vi "UHR-Fleezers Control (host) - 12.0.vi"() -> ()   [LabVIEW 2012] (continued)
            n1096 = Divide(x=w2526, y=w2525) -> (x/y=w2511:dbl[])
            n1097 = Divide(x=w2497, y=w2481) -> (x/y=w2496:dbl[])
            n1098 = Divide(x=w2495, y=w2479) -> (x/y=w2494:dbl[])
            n1099 = Build Array(w2514, w2513, w2528, w2512, w2511, w2525, w2480, w2496, w2481, w2478, w2494, w2479, w2492, w2491) -> (w2490:dbl[][])
            n1100 = Bundle("T1 Y", "T1 X", "T1 Sum", "T2 Y", "T2 X", "T2 Sum", "T1 FB Y", "T1 FB X", "T1 FB Sum", "T2 FB Y", "T2 FB X", "T2 FB Sum", "PSD X", "PSD Y Sum") -> (w2477:T40)  [unwired: 1 out]
            n1101 = To Word Integer(number=w2532) -> (16bit integer=w2476:i16[])
            n1102 = Cluster To Array(cluster=w2477) -> (array=w2523:string[])
          }
        }
      }
    }
    "AI labels" <- w1617
    n1103 = Decimate 1D Array(w1591) -> (w1615:u32[], w1559:u32[])
    n1104 = local read "DMA Update Period (s)"() -> (w1627:dbl)
    n1105 = Build Array(w1615, w1559) -> (w1685:u32[][])
    n1106 = local read "Data Period (s)"() -> (w1465:dbl)
    n1107 = local read "BD 1 Frequency 2 (MHz)"() -> (w1498:dbl)
    n1108 = local read "BD 1 Frequency 1 (MHz)"() -> (w1499:dbl)
    n1109 = Decimate 1D Array(w1506) -> (w1530:i16[], w1529:i16[], w1527:i16[], w1526:i16[])  [unwired: 9 out]
    n1110 = To Double Precision Float(number=w1685) -> (double precision float=w1686:dbl[][])
    n1111 = local read "APD Integration Time (s)"() -> (w1572:dbl)
    n1112 = Multiply(x=w1465, y="Trap Pos. Disp. Downsample") -> (x*y=w1463:dbl)
    n1113 = Divide(x=w1530, y=w1529) -> (x/y=w1531:dbl[])
    n1114 = Divide(x=w1527, y=w1526) -> (x/y=w1528:dbl[])
    n1115 = feedback #6(0.0) -> (w1544:dbl)
    n1116 = Add(x=w1627, y=w1544) -> (x+y=w1725:dbl)
    n1117 = feedback-in #6(w1725) -> ()
    n1118 = local read "AOM X Cal (nm/MHz)"() -> (w1496:dbl)
    n1119 = To Time Stamp(1:w1544) -> (0:w1543:timestamp)
    n1120 = Split 1D Array(array=w1531, index="N El. to Ave.") -> (second subarray=w1534:dbl[])  [unwired: 1 out]
    n1121 = Split 1D Array(array=w1528, index="N El. to Ave.") -> (second subarray=w1533:dbl[])  [unwired: 1 out]
    n1122 = Multiply(x=w1465, y="Trap Disp. Downsample") -> (x*y=w1545:dbl)
    "Display Period (s)" <- w1545
    n1123 = for "Trap AI" {
      tunnel: [w2275] -> w1719 mode=indexing
      tunnel: w1543 -> [w2265]
      tunnel: "Trap Disp. Downsample" -> [w2273]
      tunnel: w1618 -> [w2271] mode=indexing
      tunnel: w1465 -> [w2270]
      tunnel: w1617 -> [w2269] mode=indexing
      tunnel: w1542 -> [w2268]
      tunnel: [w2267] -> w1583 mode=indexing
      tunnel: w1545 -> [w2266]
      workers-P: _ -> [_]
      n1124 = Bundle By Name("Y"=w2271, "dt"=w2270) -> (w2272:waveform(dbl))  [unwired: 1 out]
      n1125 = Set Waveform Attribute(5:w2269, 6:w2268, 7:w2272) -> (3:w2267:waveform(dbl))  [unwired: 1 in, 2 out]
      n1126 = call "downsample 1D array - double.vi"("Ave N"=w2273, "Array In"=w2271) -> ("Array Out"=w2274:dbl[])  [unwired: 1 out]
      n1127 = Bundle By Name(cluster=w2267, "t0"=w2265, "Y"=w2274, "dt"=w2266) -> (w2275:waveform(dbl))
    }
    n1128 = Bundle("BD 1 Frequency 1 (MHz)"=w1499, "BD 1 Frequency 2 (MHz)"=w1498) -> (w1500:T41)  [unwired: 1 out]
    n1129 = call-poly <vilib>:"Mean.vi"("X"=w1533) -> ("mean"=w1521:dbl)  [unwired: 1 out]
    n1130 = call-poly <vilib>:"Mean.vi"("X"=w1534) -> ("mean"=w1522:dbl)  [unwired: 1 out]
    n1131 = Reciprocal(x=w1545) -> (1/x=→"Trap Disp. Freq. (Hz)":dbl)
    n1132 = Cluster To Array(cluster=w1500) -> (array=w1497:dbl[])
    n1133 = local read "Trap X AI1 (DMA)"() -> (w1532:T13)
    n1134 = local read "Data points/scans (MCL)"() -> (w1697:dbl)
    n1135 = To Fixed-Point(number=w1521) -> (fixed-point=w1519:fxp<+/-,16,1>)  [unwired: 1 in]
    n1136 = To Fixed-Point(number=w1522) -> (fixed-point=w1520:fxp<+/-,16,1>)  [unwired: 1 in]
    n1137 = Bundle("Trap 1 Pos.", "Trap 2 Pos.") -> (w1541:cluster{string, string})  [unwired: 1 out]
    n1138 = Bundle By Name(cluster=w1532, "Set 1"=w1520, "Set 2"=w1519) -> (→"Trap X AI1 (DMA)":T13)
    n1139 = Cluster To Array(cluster=w1541) -> (array=w1538:string[])
    n1140 = Bundle("APD 1", "APD 2") -> (w1718:cluster{string, string})  [unwired: 1 out]
    n1141 = Select(t=-1.0, s="Negate Y Axis", f=1.0) -> (s? t:f=w1482:dbl)
    n1142 = for "Trap Position" {
      tunnel: w1547 -> [w1914] mode=indexing
      tunnel: "Trap Pos. Disp. Downsample" -> [w1913]
      tunnel: w1463 -> [w1911]
      tunnel: w1543 -> [w1910]
      tunnel: w1542 -> [w1908]
      tunnel: w1538 -> [w1907] mode=indexing
      tunnel: [w1906] -> w1452 mode=indexing
      tunnel: w1497 -> [w1904] mode=indexing
      tunnel: w1496 -> [w1902]
      tunnel: w1482 -> [w1901]
      n1143 = call "downsample 1D array - double.vi"("Ave N"=w1913, "Array In"=w1914) -> ("Array Out"=w1912:dbl[])  [unwired: 1 out]
      n1144 = Subtract(x=w1912, y=w1904) -> (x-y=w1905:dbl[])
      n1145 = Multiply(x=w1902, y=w1905) -> (x*y=w1903:dbl[])
      n1146 = Multiply(x=w1901, y=w1903) -> (x*y=w1900:dbl[])
      n1147 = Bundle By Name("Y"=w1900, "dt"=w1911, "t0"=w1910) -> (w1909:waveform(dbl))  [unwired: 1 out]
      n1148 = Set Waveform Attribute(5:w1907, 6:w1908, 7:w1909) -> (3:w1906:waveform(dbl))  [unwired: 1 in, 2 out]
    }
    n1149 = Cluster To Array(cluster=w1718) -> (array=w1715:string[])
    n1150 = for "APD" {
      tunnel: w1686 -> [w2254] mode=indexing
      tunnel: w1572 -> [w2262]
      tunnel: [w2258] -> w1579 mode=indexing
      tunnel: "APD Disp. Scale" -> [w2259]
      tunnel: w1542 -> [w2257]
      tunnel: w1715 -> [w2256] mode=indexing
      tunnel: "APD Disp. Downsample" -> [w2252]
      tunnel: [w2255] -> w1714
      workers-P: _ -> [_]
      tunnel: w1543 -> [w2251]
      n1151 = call "integrate 1D array interval - double.vi"("Ave N"=w2252, "Array In"=w2254) -> ("Array Out"=w2253:dbl[])  [unwired: 1 out]
      n1152 = Multiply(x=w2262, y=w2252) -> (x*y=w2255:dbl)
      n1153 = Divide(x=w2253, y=w2259) -> (x/y=w2260:dbl[])
      n1154 = Bundle By Name("t0"=w2251, "Y"=w2260, "dt"=w2255) -> (w2261:waveform(dbl))  [unwired: 1 out]
      n1155 = Set Waveform Attribute(5:w2256, 6:w2257, 7:w2261) -> (3:w2258:waveform(dbl))  [unwired: 1 in, 2 out]
    }
    "APD Display Period (s)" <- w1714
    n1156 = Reciprocal(x=w1714) -> (1/x=→"APD Display Freq. (Hz)":dbl)
    n1157 = local read "Display Period (s)"() -> (w1603:dbl)
    n1158 = Increment(x=w1697) -> (x+1=w1698:dbl)
    n1159 = To Double Precision Float(number=w1615) -> (double precision float=w1614:dbl[])
    n1160 = Index Array(array=w1452, index=0) -> (element=w1456:waveform(dbl))
    n1161 = Index Array(array=w1452, index=1) -> (element=w1451:waveform(dbl))
    n1162 = feedback #7(w1698) -> (w1701:dbl)
    n1163 = Select(t=0, s=w1688, f=w1701) -> (s? t:f=w1694:dbl)
    n1164 = Array Size(array=w1614) -> (size(s)=w1700:i32)
    n1165 = Add(x=w1700, y=w1694) -> (x+y=w1695:dbl)
    n1166 = Unbundle By Name(w1456) -> ("Y"=w1457:dbl[])
    n1167 = feedback #8(w1615) -> (w1684:u32[])
    n1168 = Build Array (concatenate)(w1684, w1615) -> (w1681:u32[])
    n1169 = feedback #9(w1559) -> (w1578:u32[])
    n1170 = Divide(x="Bead Sep. Int. Time (s)", y=w1603) -> (x/y=w1492:dbl)
    n1171 = Build Array (concatenate)(w1578, w1559) -> (w1577:u32[])
    n1172 = Add(x=w1457, y="FB Trap Pos Offset") -> (x+y=w1455:dbl[])
    "T1 x pos data" <- w1455
    n1173 = Greater?(x=w1695, y=w1697) -> (0:w1696:bool)
    n1174 = feedback #10(w1455) -> (w1494:dbl[])
    n1175 = Build Array (concatenate)(w1455, w1494) -> (w1493:dbl[])
    n1176 = Bundle By Name(cluster=w1456, "Y"=w1455) -> (w1454:waveform(dbl))
    n1177 = Select(t=w1694, s=w1696, f=w1695) -> (s? t:f=w1693:dbl)
    n1178 = feedback-in #7(w1693) -> ()
    n1179 = Array Size(array=w1681) -> (size(s)=w1678:i32)
    n1180 = Array Size(array=w1615) -> (size(s)=w1680:i32)
    n1181 = local read "MCL Scanning"() -> (w1691:bool)
    n1182 = local read "APD Integration Time (s)"() -> (w1586:dbl)
    n1183 = Bundle(w1454, w1451) -> (w1450:cluster{waveform(dbl), waveform(dbl)})  [unwired: 1 out]
    n1184 = Build Array (concatenate)(w1579, w1719) -> (w1581:waveform(dbl)[])
    "All Signals" <- w1581
    n1185 = Split 1D Array(array=w1493, index=w1492) -> (first subarray=w1486:dbl[])  [unwired: 1 out]
    n1186 = feedback-in #10(w1486) -> ()
    n1187 = Multiply(x=w1680, y="APD Ave N") -> (x*y=w1679:dbl)
    n1188 = Greater?(x=w1678, y=w1679) -> (0:w1682:bool)
    n1189 = Not(x=w1696) -> (.not. x?=w1690:bool)
    n1190 = Cluster To Array(cluster=w1450) -> (array=w1426:waveform(dbl)[])
    "Trap Positions" <- w1426
    n1191 = To Double Precision Float(number=w1559) -> (double precision float=w1558:dbl[])
    n1192 = call-poly <vilib>:"Mean.vi"("X"=w1486) -> ("mean"=w1485:dbl)  [unwired: 1 out]
    "Mean T1 Position (nm)" <- w1485
    n1193 = Subtract(x=w1486, y=w1485) -> (x-y=w1491:dbl[])
    n1194 = Square(x=w1491) -> (x^2=w1490:dbl[])
    n1195 = And(x=w1690, y=w1691) -> (x .and. y?=w1692:bool)
    n1196 = call-poly <vilib>:"Mean.vi"("X"=w1490) -> ("mean"=w1489:dbl)  [unwired: 1 out]
    n1197 = case shown="True" w1682 {
      tunnel: w1681 -> [w2034 w2041]
      tunnel: [w2034 w2039] -> w1632
      tunnel: w1679 -> [_ w2036]
      tunnel: w1678 -> [_ w2040]
      tunnel: w1577 -> [w2033 w2038]
      tunnel: [w2033 w2035] -> w1574
      frame False {
      }
      frame True {
        n1198 = Subtract(x=w2040, y=w2036) -> (x-y=w2037:dbl)
        n1199 = Array Subset(array=w2041, index=w2037, length=w2036) -> (w2039:u32[])
        n1200 = Array Subset(array=w2038, index=w2037, length=w2036) -> (w2035:u32[])
      }
    }
    n1201 = feedback-in #8(w1632) -> ()
    n1202 = feedback-in #9(w1574) -> ()
    n1203 = Square Root(x=w1489) -> (sqrt(x)=w1488:dbl)
    n1204 = Or(x=w1692, y=w1688) -> (x .or. y?=w1689:bool)
    n1205 = Equal?(x="Tab Control 6", y=T29."High Res Display") -> (x = y?=w1621:bool)
    n1206 = Multiply(x="APD Disp. Scale", y=w1579) -> (x*y=w1588:waveform(dbl)[])
    n1207 = Multiply(x=10.0, y=w1488) -> (x*y=→"Trap 1 Position RMS (A)":dbl)
    n1208 = Multiply(x="APD Disp. Downsample", y=w1586) -> (x*y=w1584:dbl)
    n1209 = Divide(x=w1588, y=w1584) -> (x/y=w1556:waveform(dbl)[])
    n1210 = case "For displaying the high resolution display (no downsampling)" shown="True" w1621 {
      tunnel: w1583 -> [_ w1934]
      frame False {
      }
      frame True {
        n1211 = Index Array(array=w1934, index="High Res. Display") -> (element=w1935:waveform(dbl))
        n1212 = call <vilib>:"Std Deviation and Variance.vi"("X"=w1935) -> ("mean"=w1942:dbl, "standard deviation"=w1947:dbl)  [unwired: 1 in, 1 out]
        "Mean Intensity" <- w1942
        "Sigma" <- w1947
        n1213 = Subtract(x=w1935, y=w1942) -> (x-y=w1941:waveform(dbl))
        n1214 = Select(t=w1941, s="Subtract mean", f=w1935) -> (s? t:f=→"1 Channel":waveform(dbl))
        n1215 = Divide(x=w1947, y=w1942) -> (x/y=→"Sigma/Mean":dbl)
        n1216 = feedback #11(1) -> (w1936:i32)
        n1217 = Greater Or Equal?(x=w1936, y="Slow mean N ave.") -> (x >= y?=w1949:bool)
        n1218 = Increment(x=w1936) -> (x+1=w1951:i32)
        n1219 = Select(t=1, s=w1949, f=w1951) -> (s? t:f=w1938:i32)
        n1220 = feedback-in #11(w1938) -> ()
        n1221 = feedback #12() -> (w1939:waveform(dbl))  [unwired: 1 out]
        n1222 = case shown="Default" w1936 {
          tunnel: [w1954 w1957] -> w1940
          tunnel: w1939 -> [w1956 _]
          tunnel: w1935 -> [w1955 w1957]
          frame Default {
            n1223 = call-poly <vilib>:"Append Waveforms.vi"("waveform B"=w1955, "waveform A"=w1956) -> ("waveform out"=w1954:waveform(dbl))  [unwired: 1 in, 8 out]
          }
          frame 1 {
          }
        }
        n1224 = feedback-in #12(w1940) -> ()
        n1225 = case shown="True" w1949 {
          tunnel: w1940 -> [_ w1953]
          frame False {
          }
          frame True {
            n1226 = call-poly <vilib>:"Mean.vi"("X"=w1953) -> ("mean"=→"Slow mean":dbl)  [unwired: 1 out]
          }
        }
      }
    }
    n1227 = Index Array(array=w1556, index=0) -> (element=w1566:waveform(dbl))
    n1228 = Index Array(array=w1556, index=1) -> (element=w1564:waveform(dbl))
    n1229 = case "For computing FFTs for display" shown="True" "Compute FFT" {
      tunnel: w1583 -> [_ w2648]
      frame False {
      }
      frame True {
        n1230 = Build Array("FFT 1 Choice 1", "FFT 1 Choice 2", "FFT 2 Choice 1", "FFT 2 Choice 2") -> (w2641:u16[])
        n1231 = Array Size(array=w2648) -> (size(s)=w2647:i32)
        n1232 = feedback-in #13(w2641) -> ()
        n1233 = feedback #13(u16[] [100, 100, 100, 100]) -> (w2642:u16[])
        n1234 = feedback-in #14("# Spectra to Ave.") -> ()
        n1235 = feedback #14("# Spectra to Ave.") -> (w2639:dbl)
        n1236 = Not Equal?(x="# Spectra to Ave.", y=w2639) -> (x != y?=w2638:bool)
        n1237 = Not Equal?(x=w2641, y=w2642) -> (x != y?=w2640:bool)
        n1238 = feedback #15(1.0) -> (w2625:dbl)
        n1239 = Compound Arithmetic op=OR("Reset FFT", w2640, w2638) -> (w2623:bool)
        n1240 = Select(t=1.0, s=w2623, f=w2625) -> (s? t:f=w2627:dbl)
        n1241 = Greater?(x=w2627, y="# Spectra to Ave.") -> (0:w2646:bool)
        n1242 = Increment(x=w2627) -> (x+1=w2626:dbl)
        n1243 = feedback-in #15(w2626) -> ()
        n1244 = local read "DMA Update Period (s)"() -> (w2621:dbl)
        n1245 = Multiply(x="# Spectra to Ave.", y=w2621) -> (x*y=→"Ave. Time (s)":dbl)
        n1246 = Build Array(cluster{"f0":dbl, "df":dbl, "magnitude":dbl[]} {"f0"=0.0, "df"=0.0, "magnitude"=[]} ("PSD")) -> (w2630:cluster{"f0":dbl, "df":dbl, "magnitude":dbl[]}[])
        n1247 = Build Array(w2630, w2630, w2630, w2630) -> (w2632:T42)
        n1248 = feedback #16(w2632) -> (w2637:T42)
        n1249 = for {
          N: 4 -> [_]
          tunnel: w2641 -> [w2670] mode=indexing
          tunnel: w2648 -> [w2671]
          tunnel: w2647 -> [w2673]
          tunnel: w2623 -> [w2666]
          tunnel: w2646 -> [w2665]
          tunnel: "# Spectra to Ave." -> [w2664]
          tunnel: [w2663] -> w2636 mode=indexing
          tunnel: w2637 -> [w2668] mode=indexing
          tunnel: [w2667] -> w2624 mode=indexing
          tunnel: w2627 -> [w2662]
          n1250 = Less?(x=w2670, y=w2673) -> (x < y?=w2672:bool)
          n1251 = Index Array(array=w2671, index=w2670) -> (element=w2669:waveform(dbl))
          n1252 = case shown="True" w2672 {
            tunnel: w2669 -> [_ w2690]
            tunnel: w2668 -> [w2675 w2688]
            tunnel: [w2675 w2676] -> w2667
            tunnel: w2666 -> [_ w2687]
            tunnel: w2665 -> [_ w2680]
            tunnel: w2664 -> [_ w2679]
            tunnel: [cluster{"f0":dbl, "df":dbl, "magnitude":dbl[]} {"f0"=0.0, "df"=0.0, "magnitude"=[]} ("PSD") w2681] -> w2663
            tunnel: w2662 -> [_ w2678]
            frame False {
            }
            frame True {
              n1253 = call <vilib>:"Std Deviation and Variance.vi"("X"=w2690) -> ("mean"=w2691:dbl)  [unwired: 1 in, 2 out]
              n1254 = Subtract(x=w2690, y=w2691) -> (x-y=w2689:waveform(dbl))
              n1255 = xnode "Spectral Measurements"("Signals"=w2689) -> ("PSD"=w2683:cluster{"f0":dbl, "df":dbl, "magnitude":dbl[]})  [unwired: 1 in, 1 out]
              n1256 = case shown="False" w2687 {
                tunnel: w2688 -> [w2700 _]
                tunnel: [w2696 w2705] -> w2676
                tunnel: w2683 -> [w2699 w2706]
                tunnel: w2680 -> [w2698 _]
                frame False {
                  n1257 = Build Array (concatenate)(w2700, w2699) -> (w2697:cluster{"f0":dbl, "df":dbl, "magnitude":dbl[]}[])
                  n1258 = case shown="True" w2698 {
                    tunnel: w2697 -> [w2701 w2704]
                    tunnel: [w2701 w2702] -> w2696
                    frame False {
                    }
                    frame True {
                      n1259 = Delete From Array(array=w2704, index=0) -> (array with subset deleted=w2702:cluster{"f0":dbl, "df":dbl, "magnitude":dbl[]}[])  [unwired: 1 in, 1 out]
                    }
                  }
                }
                frame True {
                  n1260 = Build Array(w2706) -> (w2705:cluster{"f0":dbl, "df":dbl, "magnitude":dbl[]}[])
                }
              }
              n1261 = for {
                tunnel: w2676 -> [w2695] mode=indexing
                tunnel: [w2694] -> w2686 mode=indexing
                workers-P: _ -> [_]
                n1262 = Unbundle By Name(w2695) -> ("magnitude"=w2694:dbl[])
              }
              n1263 = Transpose 2D Array(2D array=w2686) -> (transposed array=w2685:dbl[][])
              n1264 = for {
                tunnel: w2685 -> [w2693] mode=indexing
                tunnel: [w2692] -> w2684 mode=indexing
                workers-P: _ -> [_]
                n1265 = Add Array Elements(numeric array=w2693) -> (sum=w2692:dbl)
              }
              n1266 = Select(t=w2679, s=w2680, f=w2678) -> (s? t:f=w2677:dbl)
              n1267 = Divide(x=w2684, y=w2677) -> (x/y=w2682:dbl[])
              n1268 = Bundle By Name(cluster=w2683, "magnitude"=w2682) -> (w2681:cluster{"f0":dbl, "df":dbl, "magnitude":dbl[]})
            }
          }
        }
        n1269 = case shown="True" w2623 {
          tunnel: w2624 -> [w2655 w2661]
          tunnel: [w2655 w2656] -> w2622
          frame False {
          }
          frame True {
            n1270 = Array Subset(array=w2661, index (row)=0 ("index"), length (row)=4 ("length"), index (col)=0 ("index"), length (col)=1 ("length")) -> (w2656:T42)
          }
        }
        n1271 = feedback-in #16(w2622) -> ()
        n1272 = Split 1D Array(array=w2636, index=2) -> (first subarray=→"FFT 1":cluster{"f0":dbl, "df":dbl, "magnitude":dbl[]}[], second subarray=→"FFT 2":cluster{"f0":dbl, "df":dbl, "magnitude":dbl[]}[])
      }
    }
    n1273 = case "For plotting results of scanning MCL" shown="True" w1689 {
      tunnel: w1688 -> [_ w2074]
      tunnel: w1614 -> [_ w2170]
      tunnel: w1697 -> [_ _]
      tunnel: w1583 -> [_ w2144]
      tunnel: w1558 -> [_ w2075]
      tunnel: w1557 -> [_ w2048]
      frame False {
      }
      frame True {
        w2055 = u32 0 items=["Horizontal", "Vertical", "Central", "1st Diagonal", "2nd Diagonal"] ("Type of Symmetry")
        w2083 = u32 0 items=["Horizontal", "Vertical", "Central", "1st Diagonal", "2nd Diagonal"] ("Type of Symmetry")
        w2086 = u32 0 items=["Horizontal", "Vertical", "Central", "1st Diagonal", "2nd Diagonal"] ("Type of Symmetry")
        w2115 = u32 0 items=["Horizontal", "Vertical", "Central", "1st Diagonal", "2nd Diagonal"] ("Type of Symmetry")
        n1274 = Index Array(array=w2144, index=10) -> (element=w2150:waveform(dbl))
        n1275 = Index Array(array=w2144, index=11) -> (element=w2147:waveform(dbl))
        n1276 = local read "Cycles/step (MCL)"() -> (w2100:u64)
        n1277 = Index Array(array=w2144, index="Channel") -> (element=w2146:waveform(dbl))
        n1278 = Unbundle(w2048) -> ("New Image"=w2047:T2, "New Image"=w2046:T2, "New Image"=w2045:T2, "New Image"=w2044:T2)
        n1279 = Unbundle By Name(w2150) -> ("Y"=w2102:dbl[])
        n1280 = Unbundle By Name(w2147) -> ("Y"=w2104:dbl[])
        n1281 = Unbundle By Name(w2146) -> ("Y"=w2109:dbl[])
        n1282 = call "downsample 1D array - double.vi"("Ave N"=w2100, "Array In"=w2102) -> ("Array Out"=w2101:dbl[])  [unwired: 1 out]
        n1283 = call "downsample 1D array - double.vi"("Ave N"=w2100, "Array In"=w2104) -> ("Array Out"=w2103:dbl[])  [unwired: 1 out]
        n1284 = call "downsample 1D array - double.vi"("Ave N"=w2100, "Array In"=w2109) -> ("Array Out"=w2108:dbl[])  [unwired: 1 out]
        n1285 = feedback #17(w2170) -> (w2171:dbl[])
        n1286 = Build Array (concatenate)(w2171, w2170) -> (w2152:dbl[])
        n1287 = feedback #18(w2075) -> (w2077:dbl[])
        n1288 = Build Array (concatenate)(w2077, w2075) -> (w2076:dbl[])
        n1289 = local read "Scan steps (MCL)"() -> (w2057:u64)
        n1290 = Select(t=w2170, s=w2074, f=w2152) -> (s? t:f=w2156:dbl[])
        n1291 = feedback-in #17(w2156) -> ()
        n1292 = Select(t=w2075, s=w2074, f=w2076) -> (s? t:f=w2058:dbl[])
        n1293 = feedback-in #18(w2058) -> ()
        n1294 = local read "Scan lines (y)"() -> (w2043:u64)
        n1295 = local read "N APD Samp/step"() -> (w2059:dbl)
        n1296 = feedback #19(w2101) -> (w2158:dbl[])
        n1297 = Build Array (concatenate)(w2158, w2101) -> (w2149:dbl[])
        n1298 = feedback #20(w2108) -> (w2168:dbl[])
        n1299 = Build Array (concatenate)(w2168, w2108) -> (w2167:dbl[])
        n1300 = feedback #21(w2103) -> (w2160:dbl[])
        n1301 = Build Array (concatenate)(w2160, w2103) -> (w2161:dbl[])
        n1302 = Select(t=w2101, s=w2074, f=w2149) -> (s? t:f=w2105:dbl[])
        n1303 = feedback-in #19(w2105) -> ()
        n1304 = Select(t=w2108, s=w2074, f=w2167) -> (s? t:f=w2107:dbl[])
        n1305 = feedback-in #20(w2107) -> ()
        n1306 = Select(t=w2103, s=w2074, f=w2161) -> (s? t:f=w2106:dbl[])
        n1307 = feedback-in #21(w2106) -> ()
        n1308 = Multiply(x=w2057, y=u64 2) -> (x*y=w2042:u64)
        n1309 = call "integrate 1D array interval - double.vi"("Ave N"=w2059, "Array In"=w2058) -> ("Array Out"=w2070:dbl[])  [unwired: 1 out]
        n1310 = call "integrate 1D array interval - double.vi"("Ave N"=w2059, "Array In"=w2156) -> ("Array Out"=w2155:dbl[])  [unwired: 1 out]
        n1311 = Array Size(array=w2070) -> (size(s)=w2071:i32)
        n1312 = Array Size(array=w2155) -> (size(s)=w2157:i32)
        n1313 = Multiply(x=w2043, y=w2042) -> (x*y=w2073:u64)
        n1314 = Multiply(x=w2043, y=w2042) -> (x*y=w2165:u64)
        n1315 = call-poly <vilib>:"Mean.vi"("X"=w2105) -> ("mean"=w2089:dbl)  [unwired: 1 out]
        n1316 = Subtract(x=w2073, y=w2071) -> (x-y=w2064:u64)
        n1317 = call-poly <vilib>:"Mean.vi"("X"=w2107) -> ("mean"=w2094:dbl)  [unwired: 1 out]
        n1318 = call-poly <vilib>:"Mean.vi"("X"=w2106) -> ("mean"=w2092:dbl)  [unwired: 1 out]
        n1319 = call-poly <vilib>:"Mean.vi"("X"=w2070) -> ("mean"=w2061:dbl)  [unwired: 1 out]
        n1320 = Subtract(x=w2165, y=w2157) -> (x-y=w2099:u64)
        n1321 = call-poly <vilib>:"Mean.vi"("X"=w2155) -> ("mean"=w2096:dbl)  [unwired: 1 out]
        n1322 = Initialize Array(1.0 ("element"), w2064) -> (w2060:dbl[])
        n1323 = Initialize Array(1.0 ("element"), w2099) -> (w2090:dbl[])
        n1324 = Multiply(x=w2060, y=w2061) -> (x*y=w2062:dbl[])
        n1325 = Multiply(x=w2090, y=w2092) -> (x*y=w2093:dbl[])
        n1326 = Multiply(x=w2090, y=w2094) -> (x*y=w2095:dbl[])
        n1327 = Multiply(x=w2090, y=w2089) -> (x*y=w2091:dbl[])
        n1328 = Multiply(x=w2090, y=w2096) -> (x*y=w2097:dbl[])
        n1329 = Build Array (concatenate)(w2105, w2091) -> (w2159:dbl[])
        n1330 = Build Array (concatenate)(w2107, w2095) -> (w2163:dbl[])
        n1331 = Build Array (concatenate)(w2106, w2093) -> (w2162:dbl[])
        n1332 = Build Array (concatenate)(w2070, w2062) -> (w2072:dbl[])
        n1333 = Build Array (concatenate)(w2155, w2097) -> (w2164:dbl[])
        n1334 = Reshape Array(w2159, w2043, w2042) -> (w2125:dbl[][])
        n1335 = Reshape Array(w2072, w2043, w2042) -> (w2068:dbl[][])
        n1336 = Reshape Array(w2163, w2043, w2042) -> (w2117:dbl[][])
        n1337 = Reshape Array(w2162, w2043, w2042) -> (w2132:dbl[][])
        n1338 = Reshape Array(w2164, w2043, w2042) -> (w2142:dbl[][])
        n1339 = Array Subset(array=w2132, index (col)=0 ("index"), length (col)=w2057) -> (w2137:dbl[][])  [unwired: 2 in]
        n1340 = Array Subset(array=w2132, index (col)=w2057) -> (w2135:dbl[][])  [unwired: 3 in]
        n1341 = Array Subset(array=w2117, index (col)=0 ("index"), length (col)=w2057) -> (w2123:dbl[][])  [unwired: 2 in]
        n1342 = Array Subset(array=w2117, index (col)=w2057) -> (w2121:dbl[][])  [unwired: 3 in]
        n1343 = Array Subset(array=w2068, index (col)=0 ("index"), length (col)=w2057) -> (w2067:dbl[][])  [unwired: 2 in]
        n1344 = Array Subset(array=w2068, index (col)=w2057) -> (w2065:dbl[][])  [unwired: 3 in]
        n1345 = Array Subset(array=w2142, index (col)=0 ("index"), length (col)=w2057) -> (w2141:dbl[][])  [unwired: 2 in]
        n1346 = Array Subset(array=w2142, index (col)=w2057) -> (w2139:dbl[][])  [unwired: 3 in]
        n1347 = Array Subset(array=w2125, index (col)=0 ("index"), length (col)=w2057) -> (w2130:dbl[][])  [unwired: 2 in]
        n1348 = Array Subset(array=w2125, index (col)=w2057) -> (w2128:dbl[][])  [unwired: 3 in]
        n1349 = for {
          tunnel: w2137 -> [w2179] mode=indexing
          tunnel: [w2178] -> w2136 mode=indexing
          workers-P: _ -> [_]
          n1350 = Reverse 1D Array(array=w2179) -> (reversed array=w2178:dbl[])
        }
        n1351 = for {
          tunnel: w2123 -> [w2175] mode=indexing
          tunnel: [w2174] -> w2122 mode=indexing
          workers-P: _ -> [_]
          n1352 = Reverse 1D Array(array=w2175) -> (reversed array=w2174:dbl[])
        }
        n1353 = for {
          tunnel: w2067 -> [w2173] mode=indexing
          tunnel: [w2172] -> w2066 mode=indexing
          workers-P: _ -> [_]
          n1354 = Reverse 1D Array(array=w2173) -> (reversed array=w2172:dbl[])
        }
        n1355 = for {
          tunnel: w2141 -> [w2181] mode=indexing
          tunnel: [w2180] -> w2140 mode=indexing
          workers-P: _ -> [_]
          n1356 = Reverse 1D Array(array=w2181) -> (reversed array=w2180:dbl[])
        }
        n1357 = for {
          tunnel: w2130 -> [w2177] mode=indexing
          tunnel: [w2176] -> w2129 mode=indexing
          workers-P: _ -> [_]
          n1358 = Reverse 1D Array(array=w2177) -> (reversed array=w2176:dbl[])
        }
        n1359 = Index Array(array=w2142, index (row)=0) -> (element=→"Waveform Graph":dbl[])  [unwired: 1 in]
        n1360 = Add(x=w2136, y=w2135) -> (x+y=w2134:dbl[][])
        n1361 = Add(x=w2122, y=w2121) -> (x+y=w2120:dbl[][])
        n1362 = Add(x=w2066, y=w2065) -> (x+y=w2050:dbl[][])
        n1363 = Add(x=w2140, y=w2139) -> (x+y=w2114:dbl[][])
        n1364 = Add(x=w2129, y=w2128) -> (x+y=w2127:dbl[][])
        n1365 = Divide(x=w2120, y=2) -> (x/y=w2118:dbl[][])
        n1366 = Divide(x=w2134, y=2) -> (x/y=w2079:dbl[][])
        n1367 = Divide(x=w2127, y=2) -> (x/y=w2081:dbl[][])
        n1368 = To Single Precision Float(number=w2114) -> (single precision float=w2113:sgl[][])
        n1369 = Transpose 2D Array(2D array=w2118) -> (transposed array=→"Data map":dbl[][])
        n1370 = To Single Precision Float(number=w2050) -> (single precision float=w2054:sgl[][])
        n1371 = To Single Precision Float(number=w2079) -> (single precision float=w2085:sgl[][])
        n1372 = To Single Precision Float(number=w2081) -> (single precision float=w2082:sgl[][])
        n1373 = call "IMAQ ArrayToImage"("Image Pixels (Float)"=w2113, "Image"=w2047) -> ("Image Out"=w2116:T2)  [unwired: 8 in, 1 out]
        n1374 = call "IMAQ ArrayToImage"("Image Pixels (Float)"=w2054, "Image"=w2046) -> ("Image Out"=w2056:T2)  [unwired: 8 in, 1 out]
        n1375 = call "IMAQ ArrayToImage"("Image Pixels (Float)"=w2085, "Image"=w2045) -> ("Image Out"=w2087:T2)  [unwired: 8 in, 1 out]
        n1376 = call "IMAQ ArrayToImage"("Image Pixels (Float)"=w2082, "Image"=w2044) -> ("Image Out"=w2084:T2)  [unwired: 8 in, 1 out]
        n1377 = call "IMAQ Symmetry"("Type of Symmetry"=w2115, "Image Src"=w2116) -> ("Image Dst Out"=w2111:T2)  [unwired: 3 in, 1 out]
        n1378 = call "IMAQ Symmetry"("Type of Symmetry"=w2055, "Image Src"=w2056) -> ("Image Dst Out"=w2052:T2)  [unwired: 3 in, 1 out]
        n1379 = call "IMAQ Symmetry"("Type of Symmetry"=w2086, "Image Src"=w2087) -> ("Image Dst Out"=→"Detection Laser X":T2)  [unwired: 3 in, 1 out]
        n1380 = call "IMAQ Symmetry"("Type of Symmetry"=w2083, "Image Src"=w2084) -> ("Image Dst Out"=→"Detection Laser Y":T2)  [unwired: 3 in, 1 out]
        n1381 = call "IMAQ Set Simple Calibration"("Calibration Axis Info"=T30 {"Origin Pixel"={"X"=0.0, "Y"=0.0}, "Angle Relative to Horizontal (deg)"=0.0, "Axis Reference"=0}, "Grid Descriptor"=T31 {"X Step"=0.3, "Y Step"=0.3, "Unit"=enum."Undefined"}, "Image"=w2111) -> ("Calibrated Image"=→"APD 1":T2)  [unwired: 7 in, 1 out]
        n1382 = call "IMAQ Set Simple Calibration"("Calibration Axis Info"=T30 {"Origin Pixel"={"X"=0.0, "Y"=0.0}, "Angle Relative to Horizontal (deg)"=0.0, "Axis Reference"=0}, "Grid Descriptor"=T31 {"X Step"=0.3, "Y Step"=0.3, "Unit"=enum."Undefined"}, "Image"=w2052) -> ("Calibrated Image"=→"APD 2":T2)  [unwired: 7 in, 1 out]
      }
    }
    n1383 = Subtract(x=w1564, y="APD 2 Offset") -> (x-y=w1561:waveform(dbl))
    n1384 = Subtract(x=w1566, y="APD 1 Offset") -> (x-y=w1562:waveform(dbl))
    n1385 = Index Array(array=w1581, index=3) -> (element=w1641:waveform(dbl))
    n1386 = Index Array(array=w1581, index=6) -> (element=w1638:waveform(dbl))
    n1387 = Build Array(w1562, w1561) -> (→"APD Chart":waveform(dbl)[])
    n1388 = Array Size(array=w1632) -> (size(s)=w1677:i32)
    n1389 = call <vilib>:"Std Deviation and Variance.vi"("X"=w1574) -> ("standard deviation"=w1573:dbl)  [unwired: 1 in, 2 out]
    n1390 = Add Array Elements(numeric array=w1574) -> (sum=w1576:u32)
    n1391 = Add Array Elements(numeric array=w1632) -> (sum=w1687:u32)
    n1392 = call <vilib>:"Std Deviation and Variance.vi"("X"=w1632) -> ("standard deviation"=w1631:dbl)  [unwired: 1 in, 2 out]
    n1393 = Divide(x="T1 offset_x (mV)", y=1000.0) -> (x/y=w1642:dbl)
    n1394 = Divide(x=w1573, y=w1572) -> (x/y=w1569:dbl)
    "Rate sigma (Hz) 2" <- w1569
    n1395 = Multiply(x=w1572, y=w1677) -> (x*y=w1575:dbl)
    "Int. Time (s)" <- w1575
    n1396 = Divide(x=w1576, y=w1575) -> (x/y=w1570:dbl)
    "APD 2 Rate (Hz)" <- w1570
    n1397 = Divide(x=w1687, y=w1575) -> (x/y=w1629:dbl)
    "APD 1 Rate (Hz)" <- w1629
    n1398 = Divide(x=w1631, y=w1572) -> (x/y=w1630:dbl)
    "Rate sigma (Hz)" <- w1630
    n1399 = Divide(x=w1569, y=w1570) -> (x/y=→"Sigma/Mean 2":dbl)
    n1400 = Divide(x=w1630, y=w1629) -> (x/y=→"Sigma/Mean":dbl)
    n1401 = feedback-in #22("Calibration") -> ()
    n1402 = feedback #22(u16 1 ("Calibration")) -> (w1660:u16)
    n1403 = Divide(x="T2 offset_x (mV)", y=1000.0) -> (x/y=w1640:dbl)
    n1404 = case shown="0, Default" "Calibration" {
      tunnel: "T1 alpha_x (nm/V)" -> [_ w2010 w2031]
      tunnel: "T1 kappa_x (pN/nm)" -> [_ _ w2021]
      tunnel: "T2 alpha_x (nm/V)" -> [_ w2009 w2029]
      tunnel: "T2 kappa_x (pN/nm)" -> [_ _ w2022]
      tunnel: w1641 -> [w1992 w2007 w2027]
      tunnel: w1638 -> [w1991 w2005 w2025]
      tunnel: [w1992 w2004 w2024] -> w1669
      tunnel: [w1991 w2003 w2023] -> w1668
      tunnel: ["T1 X (V)" ("Label.Text") "T1 X (nm)" ("Label.Text") "T1 X (pN)" ("Label.Text")] -> w1657
      tunnel: ["T2 X (V)" ("Label.Text") "T2 X (nm)" ("Label.Text") "T2 X (pN)" ("Label.Text")] -> w1656
      tunnel: ["Position (V)" ("Label.Text") "Position (nm)" ("Label.Text") "Force (pN)" ("Label.Text")] -> w1658
      tunnel: w1640 -> [_ w1995 w2014]
      tunnel: w1642 -> [_ w1998 w2016]
      tunnel: ["Mean (V)" ("Label.Text") "Mean (nm)" ("Label.Text") "Mean (pN)" ("Label.Text")] -> w1653
      tunnel: ["Difference (V)" ("Label.Text") "Difference (nm)" ("Label.Text") "Difference (pN)" ("Label.Text")] -> w1589
      frame 0, Default {
      }
      frame 1 {
        n1405 = Unbundle By Name(w2007) -> ("Y"=w2011:dbl[])
        n1406 = Unbundle By Name(w2005) -> ("Y"=w1996:dbl[])
        n1407 = Subtract(x=w2011, y=w1998) -> (x-y=w1999:dbl[])
        n1408 = Subtract(x=w1996, y=w1995) -> (x-y=w1997:dbl[])
        n1409 = Multiply(x=w1997, y=w2009) -> (x*y=w2006:dbl[])
        n1410 = Multiply(x=w2010, y=w1999) -> (x*y=w2008:dbl[])
        n1411 = Bundle By Name(cluster=w2005, "Y"=w2006) -> (w2003:waveform(dbl))
        n1412 = Bundle By Name(cluster=w2007, "Y"=w2008) -> (w2004:waveform(dbl))
      }
      frame 2 {
        n1413 = Unbundle By Name(w2027) -> ("Y"=w2032:dbl[])
        n1414 = Unbundle By Name(w2025) -> ("Y"=w2030:dbl[])
        n1415 = Subtract(x=w2030, y=w2014) -> (x-y=w2015:dbl[])
        n1416 = Subtract(x=w2032, y=w2016) -> (x-y=w2017:dbl[])
        n1417 = Compound Arithmetic op=MULTIPLY(w2015, w2029, w2022) -> (w2026:dbl[])
        n1418 = Compound Arithmetic op=MULTIPLY(w2021, w2031, w2017) -> (w2028:dbl[])
        n1419 = Bundle By Name(cluster=w2025, "Y"=w2026) -> (w2023:waveform(dbl))
        n1420 = Bundle By Name(cluster=w2027, "Y"=w2028) -> (w2024:waveform(dbl))
      }
    }
    n1421 = Not Equal?(x=w1660, y="Calibration") -> (x != y?=w1619:bool)
    n1422 = case shown="True" w1619 {
      tunnel: w1658 -> [_ w1985]
      tunnel: w1657 -> [_ w1984]
      tunnel: w1656 -> [_ w1983]
      tunnel: w1653 -> [_ w1982]
      tunnel: w1589 -> [_ w1981]
      frame False {
      }
      frame True {
        n1423 = property on="Force" class="WFChart (strict)"("YScale.NameLbl.Text"=w1985) -> ()  [unwired: 2 in, 2 out]
        n1424 = property on="T2 X" class="DigNum (strict)"("Caption.Text"=w1983) -> ()  [unwired: 2 in, 2 out]
        n1425 = property on="T1 X" class="DigNum (strict)"("Caption.Text"=w1984) -> ()  [unwired: 2 in, 2 out]
        n1426 = property on="Mean" class="DigNum (strict)"("Caption.Text"=w1982) -> ()  [unwired: 2 in, 2 out]
        n1427 = property on="Difference" class="DigNum (strict)"("Caption.Text"=w1981) -> ()  [unwired: 2 in, 2 out]
      }
    }
    n1428 = Unbundle By Name(w1641) -> ("Y"=w1644:dbl[])
    n1429 = Unbundle By Name(w1638) -> ("Y"=w1647:dbl[])
    n1430 = Subtract(x=w1644, y=w1642) -> (x-y=w1645:dbl[])
    n1431 = Subtract(x=w1647, y=w1640) -> (x-y=w1646:dbl[])
    n1432 = Multiply(x=w1646, y="T2 alpha_x (nm/V)") -> (x*y=w1431:dbl[])
    n1433 = Multiply(x="T1 alpha_x (nm/V)", y=w1645) -> (x*y=w1432:dbl[])
    n1434 = Not(x="Trap Trig. Fl.") -> (.not. x?=w1468:bool)
    n1435 = Multiply(x=w1668, y=-1.0) -> (x*y=w1649:waveform(dbl))
    n1436 = Subtract(x=w1432, y=w1431) -> (x-y=w1637:dbl[])
    n1437 = Unbundle By Name(w1668) -> ("Y"=w1608:dbl[])
    n1438 = Unbundle By Name(w1669) -> ("Y"=w1433:dbl[])
    n1439 = Negate(x=w1637) -> (-x=w1429:dbl[])
    n1440 = Build Array(w1669, w1649) -> (→"Force":waveform(dbl)[])
    n1441 = Subtract(x=w1429, y="Offset (nm)") -> (x-y=w1606:dbl[])
    n1442 = case shown="True" "Read Lateness and Rel Phase" {
      tunnel: w1449 -> [w1958 w1980]
      tunnel: w1448 -> [w1959 w1979]
      tunnel: [w1958 w1978] -> w1635
      tunnel: [w1959 w1977] -> w1634
      frame False {
      }
      frame True {
        n1443 = xnode "Read/Write Control"("FPGA VI Reference In"=w1980, "error in"=w1979) -> ("FPGA VI Reference Out"=w1978:T19, "error out"=w1977:errorcluster, "GI Relative phase"=→"GI relative phase":i16, "Relative phase"=→"Relative phase (AI1)":i16, "AI Late Counter"=→"Late Counter (AI1)":u16, "GI Late Counter"=→"GI Late Counter":u16, "MCL Late Counter"=→"MCL Late Counter":u16, "MCL Relative Phase"=→"Relative Phase (MCL)":i16, "APD Acq Relative Phase"=→"APD Acq Relative Phase":i16, "APD 1 Gate Relative Phase"=→"APD 1 Gate Relative Phase":i16, "APD 2 Gate Relative Phase"=→"APD 2 Gate Relative Phase":i16, "APD Acq Late Counter"=→"APD Acq Late Counter":u16, "APD 1 Gate Late Counter"=→"APD 1 Gate Late Counter":u16, "APD 2 Gate Late Counter"=→"APD 2 Gate Late Counter":u16, "Green FB Relative Phase"=→"Relative phase (Green FB)":i16, "GI Relative phase 2"=→"GI relative phase 2":i16, "GI Late Counter 2"=→"GI Late Counter 2":u16, "Trap Pos FIFO Timeout"=→"Trap Pos FIFO Timeout":u16, "Trap AI FIFO Timeout"=→"Trap AI FIFO Timeout":u16)
      }
    }
    n1444 = call-poly <vilib>:"Mean.vi"("X"=w1608) -> ("mean"=w1435:dbl)  [unwired: 1 out]
    "T2 X" <- w1435
    n1445 = Negate(x=w1608) -> (-x=w1609:dbl[])
    n1446 = call-poly <vilib>:"Mean.vi"("X"=w1433) -> ("mean"=w1436:dbl)  [unwired: 1 out]
    "T1 X" <- w1436
    n1447 = Negate(x=w1435) -> (-x=w1434:dbl)
    n1448 = Bundle By Name(cluster=w1641, "Y"=w1606) -> (w1580:waveform(dbl))
    "Bead Separation" <- w1580
    n1449 = Add(x=w1433, y=w1609) -> (x+y=w1610:dbl[])
    n1450 = Add(x=w1436, y=w1434) -> (x+y=w1655:dbl)
    n1451 = Subtract(x=w1436, y=w1434) -> (x-y=→"Difference":dbl)
    n1452 = Divide(x=w1610, y=2.0) -> (x/y=→"Vec Mean of T1 T2":dbl[])
    n1453 = Divide(x=w1655, y=2.0) -> (x/y=w1612:dbl)
    "Mean" <- w1612
    n1454 = feedback-in #23("Trap Trig. Fl.") -> ()
    n1455 = feedback #23("Trap Trig. Fl.") -> (w1466:bool)
    n1456 = And(x=w1468, y=w1466) -> (x .and. y?=w1467:bool)
    n1457 = case "If have just turned off triggering" shown="True" w1467 {
      tunnel: w1449 -> [_ w1793]
      tunnel: w1448 -> [_ w1792]
      frame False {
      }
      frame True {
        w1791 = FALSE ("FPGA Trap Trig")
        n1458 = xnode "Read/Write Control"("FPGA VI Reference In"=w1793, "error in"=w1792, "FPGA Trap Trig"=w1791) -> ("FPGA VI Reference Out"=w1790:T19, "error out"=w1789:errorcluster)
        n1459 = xnode "Read/Write Control"("FPGA VI Reference In"=w1790, "error in"=w1789, "TTrig?"=w1791) -> ()  [unwired: 2 out]
        n1460 = local write "Initializing"(FALSE ("Initializing")) -> ()
        n1461 = local write "Triggered"(FALSE ("Triggered")) -> ()
        n1462 = local write "Waiting"(FALSE ("Waiting")) -> ()
      }
    }
    n1463 = Not(x=w1466) -> (.not. x?=w1479:bool)
    n1464 = And(x="Trap Trig. Fl.", y=w1479) -> (x .and. y?=w1476:bool)
    n1465 = local read "Tether"() -> (w1613:bool)
    n1466 = Or(x=w1476, y="Reinitialize") -> (x .or. y?=w1462:bool)
    n1467 = feedback #24(w1472) -> (w1477:string)
    n1468 = Select(t=w1472, s=w1476, f=w1477) -> (s? t:f=w1471:string)
    n1469 = Select(t=w1472, s="Reinitialize", f=w1471) -> (s? t:f=w1470:string)
    n1470 = feedback #25(0) -> (w1474:i32)
    n1471 = feedback #26(w1606) -> (w1605:dbl[])
    n1472 = Build Array (concatenate)(w1606, w1605) -> (w1430:dbl[])
    n1473 = case "For determining if there is a tether still" shown="True" w1613 {
      tunnel: w1612 -> [_ w1917]
      frame False {
      }
      frame True {
        n1474 = Greater?(x="Lost Tether Alarm Threshold (pN)", y=w1917) -> (0:w1915:bool)
        n1475 = case shown="True" w1915 {
          frame False {
          }
          frame True {
            w1918 = FALSE ("Value (Signaling)")
            n1476 = flat-sequence {
              frame #0 {
                # "stop only if saving"
                n1477 = local read "Saving..."() -> (w1930:bool)
                n1478 = And(x=w1930, y="TA Cancel Save?") -> (x .and. y?=w1929:bool)
                n1479 = local write "Stop Saving"(w1929) -> ()
              }
              frame #1 {
                n1480 = case shown="True" "TA Green Off?" {
                  frame False {
                  }
                  frame True {
                    w1933 = FALSE ("Fl. Triggered...")
                    n1481 = local write "Fl. Triggered..."(w1933) -> ()
                    n1482 = property on="Green Laser ON/Interlacing" class="Bool (strict)"("Val(Sgnl)"=w1933) -> ()  [unwired: 2 in, 2 out]
                  }
                }
              }
            }
            n1483 = local read "Time tether formed"() -> (w1924:timestamp)
            n1484 = Get Date/Time In Seconds() -> (seconds since 1Jan1904=w1925:timestamp)
            n1485 = Subtract(x=w1925, y=w1924) -> (x-y=w1923:dbl)
            n1486 = Number To Decimal String(number=w1923) -> (decimal integer string=w1920:string)  [unwired: 1 out]
            n1487 = local read "Messages"() -> (w1927:string)
            n1488 = call <vilib>:"Beep.vi"() -> ()  [unwired: 3 in, 9 out]
            n1489 = Concatenate Strings("Lost tether (" ("Message to add"), w1920, " s)." ("string")) -> (w1922:string)
            n1490 = local write "Tether"(FALSE ("Tether")) -> ()
            n1491 = call "Update messages.vi"("Message to add"=w1922, "Old message string"=w1927) -> ("New message string"=w1926:string)
            n1492 = local write "Messages"(w1926) -> ()
            n1493 = property on="Fl. Triggered..." class="Bool (strict)"("Val(Sgnl)"=w1918) -> ()  [unwired: 2 in, 2 out]
            n1494 = local write "Dip for Protein"(w1918) -> ()
            n1495 = property on="Trap Pos. FB ON" class="Bool (strict)"("Val(Sgnl)"=w1918) -> ()  [unwired: 2 in, 2 out]
            n1496 = property on="Trap Trig. Fl." class="Bool (strict)"("Val(Sgnl)"=w1918) -> ()  [unwired: 2 in, 2 out]
          }
        }
      }
    }
    n1497 = case "For triggering actions based on the trap position (e.g., turning the excitation laser on if trap under feedback moves so far)" shown="True" "Trap Trig. Fl." {
      tunnel: w1457 -> [_ w1806]
      tunnel: w1470 -> [_ w1805]
      tunnel: ["" ("t") w1804] -> w1478
      tunnel: w1462 -> [_ w1803]
      tunnel: [0 ("t") w1802] -> w1475
      tunnel: w1474 -> [_ w1801]
      tunnel: w1449 -> [_ w1800]
      tunnel: w1448 -> [_ w1799]
      frame False {
      }
      frame True {
        n1498 = case shown="\"Wait for trigger\"" w1805 {
          tunnel: w1806 -> [w1823 _ _ w1871]
          tunnel: [w1820 w1852 "" ("t") w1874] -> w1804
          tunnel: w1803 -> [_ _ _ w1862]
          tunnel: [w1819 w1849 0 ("t") w1863] -> w1802
          tunnel: w1801 -> [_ w1851 _ w1869]
          tunnel: w1800 -> [w1808 w1846 _ w1865]
          tunnel: w1799 -> [w1807 w1845 _ w1864]
          frame "Wait for trigger" {
            n1499 = local read "Trap Trig. (FPGA)"() -> (w1811:bool)
            n1500 = Subtract(x=w1823, y="Mean T1 Position\nto compare (nm)") -> (x-y=w1816:dbl[])
            n1501 = call <vilib>:"Std Deviation and Variance.vi"("X"=w1816) -> ("mean"=→"mean":dbl, "standard deviation"=→"standard\ndeviation":dbl)  [unwired: 1 in, 1 out]
            n1502 = Array Max & Min(array=w1816) -> (max value=→"max value":dbl, min value=→"min value":dbl)  [unwired: 2 out]
            n1503 = Greater?(x=w1816, y="Threshold (nm)") -> (0:w1826:bool[])
            n1504 = case shown="True" w1811 {
              tunnel: w1808 -> [_ w1832]
              tunnel: w1807 -> [_ w1831]
              tunnel: [FALSE ("TTrig?") w1830] -> w1814
              frame False {
              }
              frame True {
                n1505 = xnode "Read/Write Control"("FPGA VI Reference In"=w1832, "error in"=w1831) -> ("TTrig?"=w1830:bool)  [unwired: 2 out]
              }
            }
            n1506 = Or Array Elements(Boolean array=w1826) -> (logical OR=w1813:bool)
            n1507 = Select(t=w1814, s=w1811, f=w1813) -> (s? t:f=w1812:bool)
            n1508 = Not(x=w1811) -> (.not. x?=w1810:bool)
            n1509 = And(x=w1812, y=w1810) -> (x .and. y?=w1809:bool)
            n1510 = Select(t="Triggered", s=w1812, f="Wait for trigger") -> (s? t:f=w1820:string)
            n1511 = case shown="True" w1812 {
              tunnel: [0 0] -> w1819
              tunnel: w1808 -> [_ w1837]
              tunnel: w1807 -> [_ w1836]
              frame False {
                "Waiting" <- TRUE ("Waiting")
              }
              frame True {
                n1512 = xnode "Read/Write Control"("FPGA VI Reference In"=w1837, "error in"=w1836, "TTrig?"=FALSE) -> ()  [unwired: 2 out]
                n1513 = local read "Messages"() -> (w1840:string)
                n1514 = call <vilib>:"Beep.vi"() -> ()  [unwired: 12 in]
                n1515 = call "Update messages.vi"("Message to add"="Unwinding trigger.", "Old message string"=w1840) -> ("New message string"=w1841:string)
                n1516 = local write "Messages"(w1841) -> ()
                n1517 = local write "Waiting"(FALSE ("Waiting")) -> ()
                "Triggered" <- TRUE ("Triggered")
              }
            }
            n1518 = case "Only need to turn on laser if host triggered" shown="True" w1809 {
              frame False {
              }
              frame True {
                n1519 = property on="Green Laser ON/Interlacing" class="Bool (strict)"("Val(Sgnl)"=TRUE ("Value (Signaling)")) -> ()  [unwired: 2 in, 2 out]
              }
            }
          }
          frame "Triggered" {
            n1520 = local read "Trap Trig. (FPGA)"() -> (w1848:bool)
            n1521 = Increment(x=w1851) -> (x+1=w1849:i32)
            n1522 = Greater Or Equal?(x=w1849, y="Fl. ON time (n)") -> (x >= y?=w1847:bool)
            n1523 = Select(t="Wait for trigger", s=w1847, f="Triggered" ("t")) -> (s? t:f=w1852:string)
            n1524 = And(x=w1847, y=w1848) -> (x .and. y?=w1844:bool)
            n1525 = case shown="True" w1844 {
              tunnel: w1846 -> [_ w1856]
              tunnel: w1845 -> [_ w1855]
              frame False {
              }
              frame True {
                n1526 = xnode "Read/Write Control"("FPGA VI Reference In"=w1856, "error in"=w1855, "FPGA Trap Trig"=TRUE) -> ()  [unwired: 2 out]
              }
            }
            n1527 = case shown="True" w1847 {
              frame False {
              }
              frame True {
                w1858 = FALSE ("Value (Signaling)")
                n1528 = local write "Triggered"(w1858) -> ()
                n1529 = local write "Waiting"(TRUE ("Waiting")) -> ()
                n1530 = property on="Green Laser ON/Interlacing" class="Bool (strict)"("Val(Sgnl)"=w1858) -> ()  [unwired: 2 in, 2 out]
              }
            }
          }
          frame "Do nothing" {
          }
          frame "Initialize", Default {
            n1531 = Increment(x=w1869) -> (x+1=w1873:i32)
            n1532 = Select(t=1, s=w1862, f=w1873) -> (s? t:f=w1863:i32)
            n1533 = feedback #27(w1871) -> (w1877:dbl[])
            n1534 = Build Array (concatenate)(w1871, w1877) -> (w1870:dbl[])
            n1535 = Greater Or Equal?(x=w1863, y="Wait to get offset (n)") -> (x >= y?=w1866:bool)
            n1536 = Select(t=w1871, s=w1862, f=w1870) -> (s? t:f=w1872:dbl[])
            n1537 = feedback-in #27(w1872) -> ()
            n1538 = call-poly <vilib>:"Mean.vi"("X"=w1872) -> ("mean"=w1867:dbl)  [unwired: 1 out]
            n1539 = local write "Mean T1 Position\nto compare (nm)"(w1867) -> ()
            n1540 = case shown="True" w1862 {
              tunnel: w1865 -> [_ w1883]
              tunnel: w1864 -> [_ w1882]
              frame False {
              }
              frame True {
                w1879 = FALSE ("FPGA Trap Trig")
                n1541 = xnode "Read/Write Control"("FPGA VI Reference In"=w1883, "error in"=w1882, "FPGA Trap Trig"=w1879) -> ("FPGA VI Reference Out"=w1881:T19, "error out"=w1880:errorcluster)
                n1542 = xnode "Read/Write Control"("FPGA VI Reference In"=w1881, "error in"=w1880, "TTrig?"=w1879) -> ()  [unwired: 2 out]
              }
            }
            n1543 = Select(t="Wait for trigger", s=w1866, f="Initialize") -> (s? t:f=w1874:string)
            n1544 = case shown="True" w1866 {
              tunnel: w1867 -> [_ w1886]
              tunnel: w1865 -> [_ w1895]
              tunnel: w1864 -> [_ w1894]
              frame False {
                n1545 = local write "Waiting"(FALSE ("Waiting")) -> ()
                "Initializing" <- TRUE ("Initializing")
              }
              frame True {
                n1546 = local read "Threshold (nm)"() -> (w1898:dbl)
                n1547 = local read "AOM X Cal (nm/MHz)"() -> (w1897:dbl)
                n1548 = Add(x=w1886, y=w1898) -> (x+y=w1899:dbl)
                n1549 = Divide(x=w1899, y=w1897) -> (x/y=w1896:dbl)
                n1550 = call "IR AOM freq to word.vi"("Frequency In (MHz)"=w1896) -> ("Frequency Word Out (double)"=w1893:dbl)
                n1551 = local write "Initializing"(FALSE ("Initializing")) -> ()
                n1552 = local write "Waiting"(TRUE ("Waiting")) -> ()
                n1553 = To Quad Integer(1:w1893) -> (0:w1892:i64)
                n1554 = xnode "Read/Write Control"("FPGA VI Reference In"=w1895, "error in"=w1894, "FPGA TTrig Thresh"=w1892) -> ("FPGA VI Reference Out"=w1889:T19, "error out"=w1888:errorcluster)
                n1555 = xnode "Read/Write Control"("FPGA VI Reference In"=w1889, "error in"=w1888, "FPGA Trap Trig"=TRUE) -> ()  [unwired: 2 out]
              }
            }
          }
        }
      }
    }
    n1556 = feedback-in #24(w1478) -> ()
    n1557 = feedback-in #25(w1475) -> ()
    n1558 = Split 1D Array(array=w1430, index=w1492) -> (first subarray=w1602:dbl[])  [unwired: 1 out]
    n1559 = feedback-in #26(w1602) -> ()
    n1560 = call-poly <vilib>:"Mean.vi"("X"=w1602) -> ("mean"=w1601:dbl)  [unwired: 1 out]
    "Bead Mean (nm)" <- w1601
    n1561 = Subtract(x=w1602, y=w1601) -> (x-y=w1600:dbl[])
    n1562 = Square(x=w1600) -> (x^2=w1599:dbl[])
    n1563 = call-poly <vilib>:"Mean.vi"("X"=w1599) -> ("mean"=w1598:dbl)  [unwired: 1 out]
    n1564 = Square Root(x=w1598) -> (sqrt(x)=w1597:dbl)
    n1565 = Multiply(x=10.0, y=w1597) -> (x*y=→"RMS (Ang)":dbl)
    n1566 = xnode ("Read/Write Control")("FPGA VI Reference In"=w1635, "error in"=w1634) -> ("FPGA VI Reference Out"=w1460:T19, "error out"=w1459:errorcluster, "AI2 Y Sum Set 1"=w1733:i16, "AI2 Y Sum Set 2"=w1732:i16, "AI1 X Set 1"=w1524:fxp<+/-,16,1>, "AI1 X Set 2"=w1523:fxp<+/-,16,1>, "Trap Pos FB Int Signal"=→"Trap Pos FB Int Signal":fxp<+/-,24,9>, "Trap Pos FB Int-Norm Signal"=→"Trap Pos FB Int-Norm Signal":fxp<+/-,16,1>, "Trap Pos FB Action"=w1517:i64, "Scanning"=→"AOD Scanning":bool, "Scan I"=→"AOD Scan I":u64, "Scanning MCL"=w1735:bool, "Scan I (MCL)"=→"MCL Scan I":u64, "Green FB Sum"=w1672:i16, "Trap Pos FB Action"=w1447:i64, "TTrig Fin Thresh"=w1443:i64)
    "MCL Scanning" <- w1735
    "Trap Pos FB Action" <- w1517
    n1567 = local read "FB Trig Integrate"() -> (w1441:u32)
    n1568 = Divide(x=w1672, y=3276.7) -> (x/y=→"Green laser plot" →"Green laser intensity (V)":dbl)
    n1569 = Divide(x=w1447, y=w1441) -> (x/y=w1440:dbl)
    "TTrig Sig (Int)" <- w1440
    n1570 = Divide(x=w1443, y=w1441) -> (x/y=w1438:dbl)
    "TTrig Fin Thresh (Int)" <- w1438
    n1571 = local read "AOM X Cal (nm/MHz)"() -> (w1446:dbl)
    n1572 = local read "AI2 (V)"() -> (w1734:cluster{"Set 1":dbl, "Set 2":dbl})
    n1573 = Bundle By Name(cluster=w1734, "Set 1"=w1733, "Set 2"=w1732) -> (w1730:cluster{"Set 1":dbl, "Set 2":dbl})
    n1574 = Divide(x=w1517, y=327.67) -> (x/y=→"Action (%)":dbl)
    n1575 = local read "Trap X (AI1)"() -> (w1537:T10)
    n1576 = call "IR AOM word double to freq.vi"("Frequency Word In (double)"=w1438) -> ("Frequency Out (MHz)"=w1437:dbl)
    n1577 = call "IR AOM word double to freq.vi"("Frequency Word In (double)"=w1440) -> ("Frequency Out (MHz)"=w1439:dbl)
    n1578 = Divide(x=w1730, y=3276.7) -> (x/y=w1729:cluster{"Set 1":dbl, "Set 2":dbl})
    n1579 = Multiply(x=w1439, y=w1446) -> (x*y=w1445:dbl)
    "TTrig Sig (nm)" <- w1445
    n1580 = Multiply(x=w1437, y=w1446) -> (x*y=w1444:dbl)
    "TTrig Fin Thresh (nm)" <- w1444
    n1581 = local write "AI2 (V)"(w1729) -> ()
    n1582 = Bundle(cluster=w1537, "Trap 1"=w1524, "Trap 2"=w1523) -> (→"Trap X (AI1)":T10)
    n1583 = Bundle(w1445, w1444) -> (→"TTrig":cluster{dbl, dbl})  [unwired: 1 in]
    n1584 = flat-sequence "To save data" {
      tunnel: [w2754] -> w1753
      tunnel: [w2755] -> w1752
      tunnel: w1703 -> [w2748]
      tunnel: w1465 -> [w2752]
      tunnel: ["Save Calibration"] -> w1726
      tunnel: w1723 -> [w2751]
      tunnel: [w2744] -> w1722
      tunnel: [w2741] -> w1721
      tunnel: [w2738] -> w1720
      tunnel: w1702 -> [w2740]
      tunnel: w1617 -> [w2734]
      tunnel: [w2734] -> w1616
      tunnel: ["Start Saving"] -> w1582
      tunnel: [w2728] -> w1505
      tunnel: [w2727] -> w1504
      tunnel: w1753 -> [w2990]
      tunnel: w1752 -> [w2989]
      tunnel: w1506 -> [w2988]
      tunnel: w1726 -> [w2987]
      tunnel: w1722 -> [w2985]
      tunnel: w1721 -> [w2984]
      tunnel: w1720 -> [w2983]
      tunnel: w1591 -> [w2982]
      tunnel: w1627 -> [w2981]
      tunnel: w1616 -> [w2980]
      tunnel: w1582 -> [w2979]
      tunnel: w1580 -> [w2978]
      tunnel: w1556 -> [w2977]
      tunnel: w1505 -> [w2976]
      tunnel: w1504 -> [w2975]
      tunnel: w1503 -> [w2974]
      tunnel: w1426 -> [w2973]
      frame #0 {
        n1585 = Or(x="Save N Sets", y="Start Saving") -> (x .or. y?=w2735:bool)
        n1586 = To Double Precision Float(number=w2751) -> (double precision float=w2745:dbl)
        n1587 = Build Array(w2735, "Save Calibration", w2748, w2740) -> (w2750:bool[])
        n1588 = Compound Arithmetic op=OR("Save Calibration", w2748, w2735, w2740) -> (w2753:bool)
        n1589 = Boolean Array To Number(Boolean array=w2750) -> (number=w2747:u32)
        n1590 = feedback #28(FALSE ("Save APD Data\nwith Trap Data")) -> (w2729:bool)
        n1591 = feedback #29(refnum<k0> refnum) -> (w2756:refnum<file>)
        n1592 = feedback #30(refnum<k0> refnum) -> (w2731:refnum<file>)
        n1593 = feedback #31(FALSE ("Save APD Data\nwith Trap Data")) -> (w2739:bool)
        n1594 = feedback #32(refnum<k0> refnum) -> (w2742:refnum<file>)
        n1595 = feedback #33(0) -> (w2758:i32)
        n1596 = feedback #34() -> (w2746:u32)  [unwired: 1 out]
